vi "CAN1.vi"() -> ()   [LabVIEW 2020]
uses:
  Global_Variable/Global.vi
  Global_Variable/A180648.vi
  Libraries/ZLG_CAN/ZLG_CAN.lvlib
panel:
  out "error out":errorcluster caption="错误输出"
  in  "CAN 通道":u32(ring)=1 items=["0", "1"]
  in  "索引":u32(ring) items=["0", "1", "2", "3", "4", "5", "6", "7", "8"]
  in  "设备类型":u32(ring)=27 items=["PCI5121"=1, "PCI9810"=2, "USBCAN1"=3, "USBCAN2"=4, "PCI9820"=5, "PCI5110"=7, "PC104CAN"=11, "CANETUDP"=12, "PCI9840B"=14, "PC104C2"=15, "PCI9820I"=16, "CANETTCP"=17, "PCIE9221"=24, "PCI5010U"=19, "USBCAN_E_U"=20, "USBCAN_2E_U"=21, "PCI5020U"=22, "PCIE9120I"=27, "PCIE9110I"=28, "PCIE9140I"=29]
  in  "Stop":bool
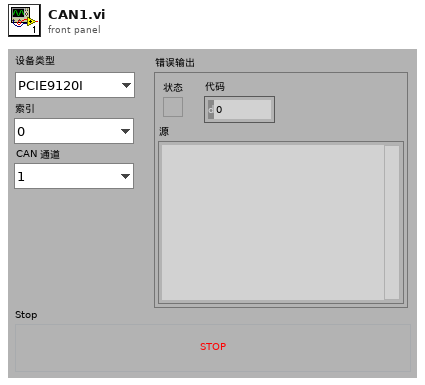
[diagram p1: front panel]
types:
  T1 = cluster{"波特率":u32, "ID":u32, "帧类型":enum8{"标准帧", "扩展帧"}, "帧格式":enum16{"数据帧", "远程帧"}, "周期(ms)":u32}
  T2 = typedef "ZLG_CAN.lvlib/Start_CAN (Reply Payload)--cluster.ctl" = cluster{"Success":bool, "Start_CAN_error":errorcluster}
  T3 = cluster{u8, u8, "y":u8, "y":u8, "y":u8, "y":u8, "y":u8, "y":u8}
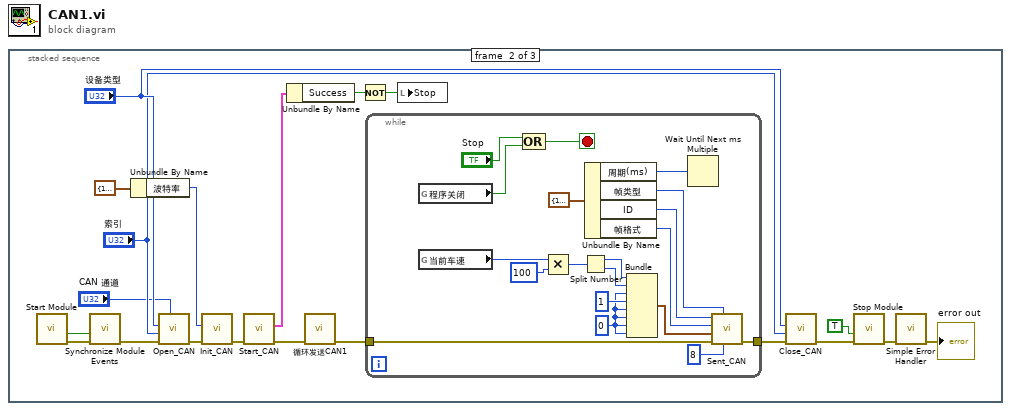
[diagram p0: block diagram]
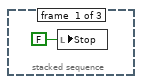
[diagram p2: hidden frame]
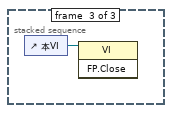
[diagram p3: hidden frame]
diagram:
  n1 = stacked-sequence {
    frame #0 {
      n2 = local write "Stop"(FALSE ("Stop")) -> ()
    }
    frame #1 {
      n3 = call "Start Module.vi"() -> ("error out"=w21:errorcluster, "Wait for Event Sync?"=w20:bool)  [unwired: 8 in, 2 out]
      n4 = call "Synchronize Module Events.vi"("error in (no error)"=w21, "Wait for Event Sync?"=w20) -> ("error out"=w19:errorcluster)  [unwired: 9 in]
      n5 = Unbundle By Name(T1 {"波特率"=11, "ID"=745, "帧类型"=enum."标准帧", "帧格式"=enum."数据帧", "周期(ms)"=10} ("CAN Info")) -> ("波特率"=w11:u32)
      n6 = call "Open_CAN.vi"("CAN 通道"="CAN 通道", "error in (no error)"=w19, "索引"="索引", "设备类型"="设备类型") -> ("error out"=w16:errorcluster)  [unwired: 7 in]
      n7 = call "Init_CAN.vi"("error in (no error)"=w16, "波特率"=w11) -> ("error out"=w12:errorcluster)  [unwired: 9 in]
      n8 = call "Start_CAN.vi"("error in (no error)"=w12) -> ("error out"=w10:errorcluster, "Reply Payload"=w14:T2)  [unwired: 8 in, 1 out]
      n9 = Unbundle By Name(w14) -> ("Success"=w13:bool)
      n10 = call "循环发送CAN1.vi"("错误输入"=w10) -> ("错误输出"=w9:errorcluster)  [unwired: 10 in]
      n11 = Not(x=w13) -> (.not. x?=w8:bool)
      n12 = while {
        tunnel: w9 -> [w40]
        tunnel: [w39] -> w5
        stop <- w37 stop-if-true
        w23 = u8 0 ("y")
        n13 = global read "Global.vi" "程序关闭"() -> (w36:bool)
        n14 = global read "A180648.vi" "当前车速"() -> (w24:u16)
        n15 = Compound Arithmetic op=OR ("复合运算")("Stop", w36) -> (w37:bool)
        n16 = Multiply(x=w24, y=u16 100) -> (x*y=w34:u16)
        n17 = Split Number(x=w34) -> (hi(x)=w33:u8, lo(x)=w32:u8)
        n18 = Unbundle By Name(T1 {"波特率"=11, "ID"=745, "帧类型"=enum."标准帧", "帧格式"=enum."数据帧", "周期(ms)"=10} ("CAN Info")) -> ("周期(ms)"=w28:u32, "帧类型"=w26:enum8{"标准帧", "扩展帧"}, "ID"=w25:u32, "帧格式"=w27:enum16{"数据帧", "远程帧"})
        n19 = Bundle(w33, w32, "y"=w23, "y"=u8 1, "y"=w23, "y"=w23, "y"=w23, "y"=w23) -> (w30:T3)  [unwired: 1 in]
        n20 = Wait Until Next ms Multiple(millisecond multiple=w28) -> ()  [unwired: 1 out]
        n21 = call "Sent_CAN.vi"("帧长度"=u8 8, "帧类型"=w26, "error in (no error)"=w40, "帧数据"=w30, "帧格式"=w27, "ID"=w25) -> ("error out"=w39:errorcluster)  [unwired: 5 in]
      }
      n22 = local write "Stop"(w8) -> ()
      n23 = call "Close_CAN.vi"("error in (no error)"=w5, "索引"="索引", "设备类型"="设备类型") -> ("error out"=w6:errorcluster)  [unwired: 8 in]
      n24 = call "Stop Module.vi"("error in (no error)"=w6, "Wait for Module to Stop? (F)"=TRUE) -> ("error out"=w4:errorcluster)  [unwired: 9 in]
      n25 = call <vilib>:"Simple Error Handler.vi"("error in (no error)"=w4) -> ("error out"=→"error out":errorcluster)  [unwired: 4 in, 4 out]
    }
    frame #2 {
      n26 = control-ref of="本VI"() -> (w41:refnum<vi>)
      n27 = invoke class="VI" method="FP.Close"(reference=w41) -> ()  [unwired: 2 in, 3 out]
    }
  }
